vi "traceFileIO_writeToFile_multiple.vi"(0 "reference in":refnum<class "OSA.lvclass">, 1 "Path":path, 3 "dataType":T2, 4 "traces idx":u32[](array[numeric]), 5 "error in (no error)":errorcluster, 7 "dialog (empty path)":bool) -> (13 "traces idx global":u32[](array[numeric]), 14 "reference out":refnum<class "OSA.lvclass">, 15 "actual path":path, 17 "cancelled":bool, 19 "error out":errorcluster)   [LabVIEW 2010, in "OSA.lvclass"]
doc: "Read several spectrum or interferogram data from traces, (FTSLib.dll allocated), and store in a single spf2 file."
uses:
  OSA.lvclass
  typeDef/acq_dataType.ctl
  typeDef/trace_properties_ui.ctl
  FTSLib.dll
  OSA20X_misc.lvlib
panel:
  in  "property":T1
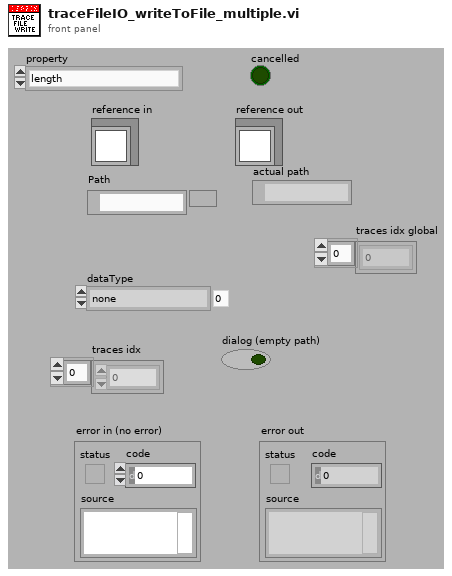
[diagram p1: front panel]
types:
  T1 = typedef "OSA.lvclass/trace_properties_ui.ctl" = enum16{"length", "type", "acquisitionMode", "xValueFormat", "date", "time", "averageNum", "smoothType", "igramSmoothType", "phaseCorrection", "apodisation", "__allocatedLengthI", "__allocatedLengthx", "adcBits", "sensitivityMode", "resolutionMode", "rollingAverage", "samplesPerReference", "air_measureOption", "interferogramProperty", "all_uiProperties"}
  T2 = typedef "OSA.lvclass/acq_dataType.ctl" = enum16{"none", "interferogram", "spectrum"}
  T3 = enum16{"SPC", "CSV", "SPF2", "TXT", "MAT_V5", "CSV_ZIP", "TXT_ZIP", "JCAMPDX"}
  T4 = typedef "OSA.lvclass/ObjectAttributes.ctl" = cluster{"Stop":bool, "dataType":T2, "spectrometerIdx":u16, "buffer size interferogram":i32, "interferogram":cluster{"new":bool, "plot_x_ min":sgl, "plot_x_max":sgl, "plot_y_min":sgl, "plot_y_max":sgl, "Graph Intrfrgrm":T5, "timeStamp":u32, "signal (%)":dbl, "traces":cluster{"idx":u32, "broadBand":bool, "monoChromatic":bool, "peakToPeakSignal":dbl, "peakToPeakPos":dbl}[], "traces idx last":i32}, "spectrum":cluster{"new":bool, "plot_x_min":sgl, "plot_x_max":sgl, "plot_unit_x":T6, "plot_unit_y":T7, "plot_y_min":sgl, "plot_y_max":sgl, "Graph Spectrum":T5, "timeStamp":u32, "X_VAL_OPTIONS":enum16{"MIN_MAX", "ARRAY"}, "traces":cluster{"idx":u32}[], "traces idx last":i32}, "Thorlabs_OSA_64.lvclass:queue_action.ctlqueue ref":refnum<queue>, "action":T8, "plot zoom step":dbl, "buffer semaphore":T9, "acq stopped":bool, "dataType active":T2, "temperature (degr C)":sgl, "pressure (hPa)":sgl, "rel humidity (%)":sgl, "settings":cluster{"resolution":T10, "sensitivity":T11, "Average":bool, "average nr":u32, "apodisation":T12, "acq delay (ms)":u32, "airMesure":T13, "wmtr on":bool, "intfgrm_smooth_width":u16, "intfgrm_smooth_nrOfPasses":u16, "intfgrm_smooth":T14, "phaseCorrection":T15, "zeroFill":u8, "spectr_smooth":T14, "spectr_smooth_width":u16, "spectr_smooth_nrOfPasses":u16, "resolution (/cm)":sgl, "REF wavelength, (nm)":dbl, "gain_idx":u16, "gainAuto":bool, "gain_relative":dbl, "PD sensitivity mode":T16, "PD senseMode implemented":bool, "SensorTemperature implemented":bool, "SensorPressure implemented":bool, "SensorHumidity implemented":bool}, "peaks position":sgl[], "peaks width":sgl[], "peaks height":sgl[], "peaks max nr":u32, "peaks latest nr":i32, "peaks new":bool, "power":dbl, "power new":bool, "path":string, "wavelength (WNr)":dbl, "wavelength new":bool, "buffer size spectrum":i32, "status":string, "VI reference":refnum<vi>, "funcPointer":u64, "libraryPointer":u64, "singleAcquisition":bool, "coherenceLength (cm)":dbl, "coherenceLength new":bool, "spectrometer model":string, "spectrometer serial nr":string, "peaks thld left":sgl[], "peaks thld right":sgl[], "coherenceLength error (cm)":dbl, "ADC bits":u16, "peaks position centroid":sgl[], "peaks height centroid":sgl[], "OSA series":T17, "channel index spectrum":u16, "spectrometer rangeLow, (/cm)":dbl, "spectrometer rangeHigh, (/cm)":dbl, "channel index interferogram":u16}
  T5 = typedef "OSA.lvclass/graph_intensity.ctl" = refnum<vi>
  T6 = typedef "OSA.lvclass/spectrum_x_unit.ctl" = enum16{"wavenr/cm", "THz", "eV", "nm_air", "nm_vac"}
  T7 = typedef "OSA.lvclass/y_unit.ctl" = enum16{"ADC counts", "dBm pwr absolute", "dBm pwr density", "mW pwr absolute", "mW pwr density"}
  T8 = typedef "OSA.lvclass/queue_action.ctl" = enum16{"none", "stop", "GUI_plotInterferogram", "GUI_plotSpectrum", "GUI_plotInterferogramRescale", "GUI_plotSpectrumRescale", "GUI_plotInterferogramReset", "GUI_plotSpectrumReset", "GUI_plotInterferogramAutoScaleY", "GUI_plotSpectrumAutoScaleY", "GUI_plotInterferogramZoomOut", "GUI_plotSpectrumZoomOut", "GUI_plotInterferogramPane", "GUI_plotSpectrumPane", "GUI_plotInterferogramZoomMouse", "GUI_plotSpectrumZoomMouse", "ENVIRONMENT temperature", "ENVIRONMENT pressure", "MODE_resolution set", "MODE_resolution get", "MODE_sensitivity set", "MODE_sensitivity get", "MODE_PDTemperature set", "MODE_PDTemperature get", "REBOOT/RESET firmware", "ACQASYNC_acquireSingleSpectrum", "ACQASYNC_continuous start", "ACQASYNC_continuous stop\n", "ACQASYNC_get last interferogram", "ACQASYNC_get last spectrum", "ACQASYNC_get last waveNr", "ACQOPT_interferogram smoothing set", "ACQOPT_interferogram smoothing get", "ACQOPT_spectrum smoothing set", "ACQOPT_spectrum smoothing get", "ACQOPT_apodisation type set", "ACQOPT_apodisation type get", "ACQOPT_phase correction type set", "ACQOPT_phase correction type get", "ACQOPT_acqIntervall_set", "ACQOPT_acqIntervall_get", "ACQOPT_average spectrum set", "ACQOPT_average spectrum get", "ACQOPT_rolling average set", "ACQOPT_rolling average get", "ACQOPT_zero fill factor set", "ACQOPT_zero fill factor get", "ACQOPT_cycle counting set", "ACQOPT_cycle counting get", "ACQOPT_air measure option set", "ACQOPT_air measure option get", "ACQOPT_gainLevel auto get", "ACQOPT_gainLevel auto set", "ACQOPT_gainLevel get", "ACQOPT_gainLevel set", "ACQOPT_getAll", "INSTRUMENT_PROPERTY_range_WaveNr_min", "INSTRUMENT_PROPERTY_range_WaveNr_max", "INSTRUMENT_PROPERTY_reference_wavelength_cm^-1", "INSTRUMENT_PROPERTY_samplesPerRefPeriod", "INSTRUMENT_PROPERTY_resolution_waveNrPercm", "INSTRUMENT_PROPERTY_availableGainLevels", "INSTRUMENT_PROPERTY_status", "CONVERT", "ANALYSE_POWER", "ANALYSE_PEAKS", "ANALYSE_WAVELENGTH", "ANALYSE_SPECTRUM", "ANALYSE_INTERFEROGRAM", "ANALYSE_COHERENCE_LENGTH", "MATH", "MATH_power", "MATH_peaks", "FILE", "miscellaneous"}
  T9 = typedef "Semaphore RefNum" = refnum<k1>
  T10 = typedef "OSA.lvclass/resolution.ctl" = enum16{"low", "high"}
  T11 = typedef "OSA.lvclass/sensitivityMode.ctl" = enum16{"low", "low medium", "high medium", "high"}
  T12 = typedef "OSA.lvclass/apodisation.ctl" = enum16{"NONE", "NORTON_BEER_WEAK", "NORTON_BEER_MEDIUM", "NORTON_BEER_STRONG", "TRIANGULAR", "COSINE", "HANN", "HAMMING", "BLACKMANHARRIS3", "BLACKMANHARRIS4", "GAUSSIAN"}
  T13 = typedef "OSA.lvclass/airMeasure.ctl" = enum16{"TEMPERATURE", "PRESSURE"}
  T14 = typedef "OSA20X_misc.lvlib/interferogram_smoothing.ctl" = enum16{"NONE", "BINOMIAL", "SAVITSKY_GOLAY", "FOURIER", "MOVING_AVERAGE", "GAUSSIAN"}
  T15 = typedef "OSA.lvclass/phaseCorrection.ctl" = enum16{"NONE", "MERTZ", "FORMAN", "MERTZ_FILE", "FORMAN_FILE", "FUTURE COMP."}
  T16 = typedef "OSA20X_misc.lvlib/PDTemperatureMode.ctl" = enum16{"cool: better sensitivity/noise floor", "warm: extended wl range"}
  T17 = typedef "OSA.lvclass/OSA_series.ctl" = enum16{"OSA200", "OSA300", "UNKNOWN"}
  T18 = cluster{"idx":u32, "broadBand":bool, "monoChromatic":bool, "peakToPeakSignal":dbl, "peakToPeakPos":dbl}[]
  T19 = cluster{"property":string, "property value":u32}[]
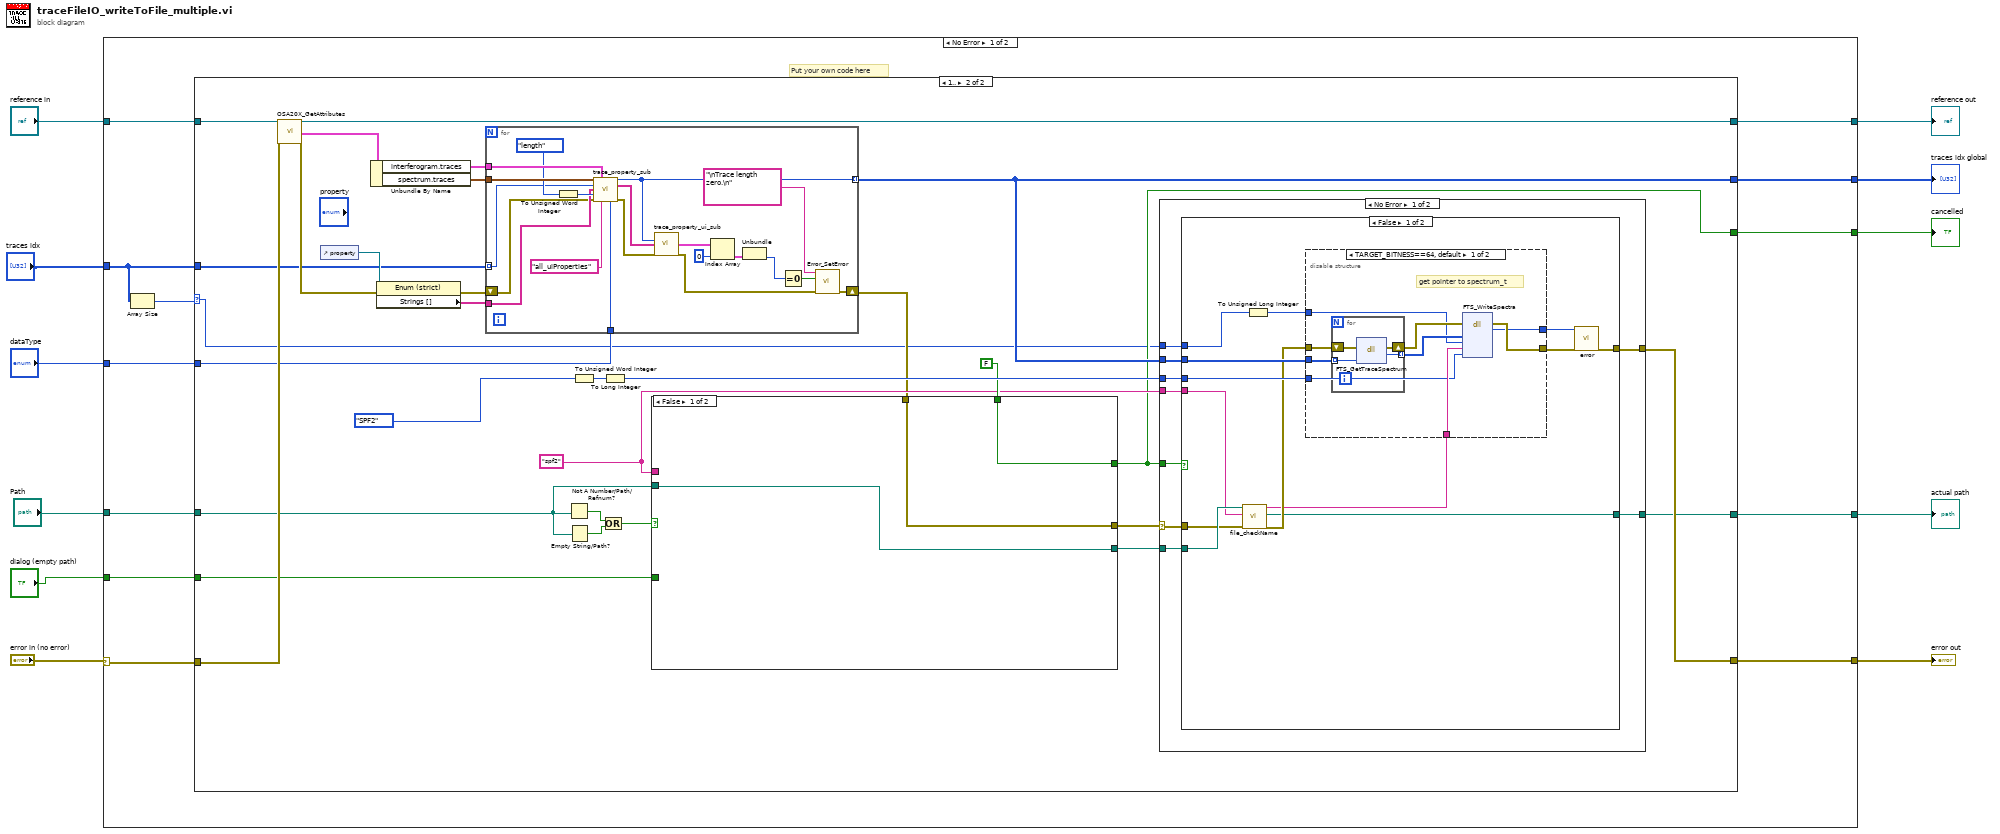
[diagram p0: block diagram]
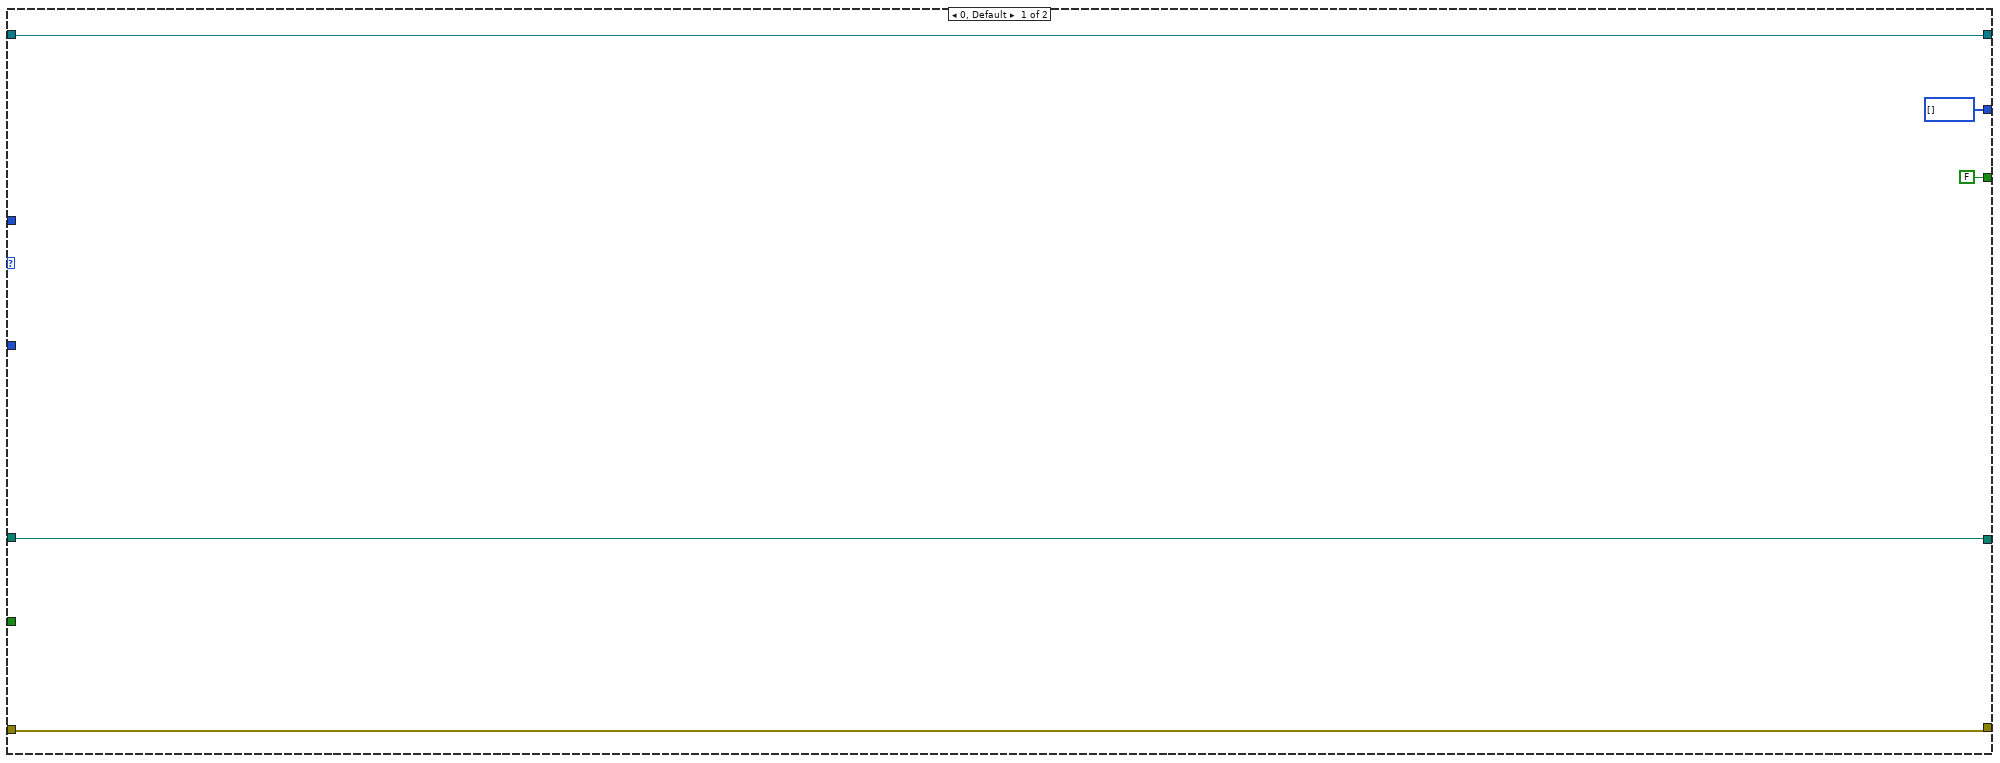
[diagram p2: hidden frame]
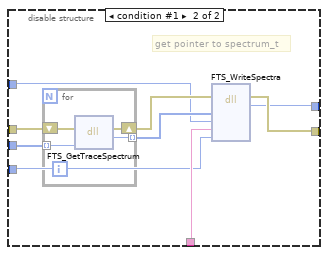
[diagram p3: hidden frame]
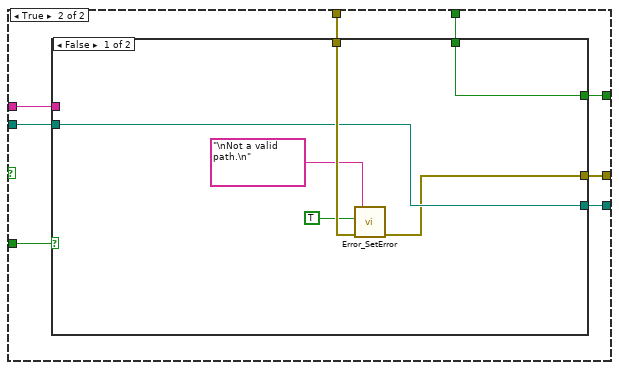
[diagram p6: hidden frame]
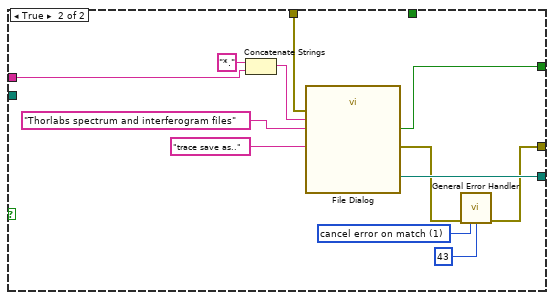
[diagram p7: hidden frame]
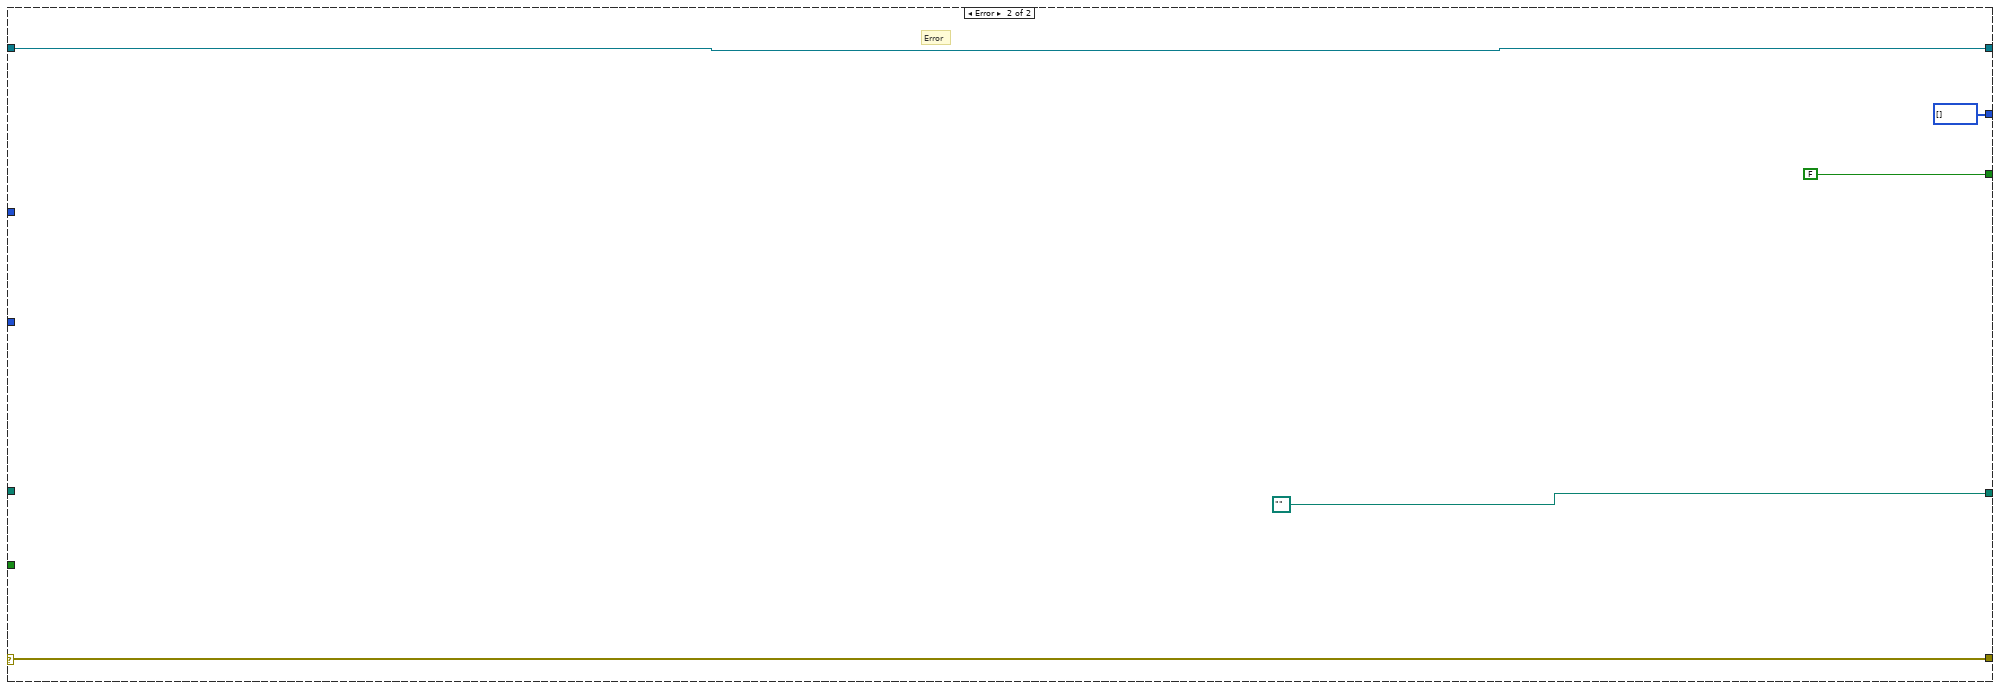
[diagram p8: hidden frame]
diagram:
  n1 = case shown="No Error" "error in (no error)" {
    selector: "error in (no error)" -> [w23 w164]
    tunnel: [w19 w164] -> w11
    tunnel: "reference in" -> [w22 w163]
    tunnel: [w21 w163] -> w8
    tunnel: "dataType" -> [w15 _]
    tunnel: "traces idx" -> [w12 _]
    tunnel: [w16 u32[] []] -> w6
    tunnel: "Path" -> [w20 _]
    tunnel: "dialog (empty path)" -> [w18 _]
    tunnel: [w17 path "" ("selected path")] -> w3
    tunnel: [w14 FALSE ("cancelled")] -> w2
    frame No Error {
      # "Put your own code here"
      n2 = Array Size(array=w12) -> (size(s)=w13:i32)
      n3 = case shown="1.." w13 {
        selector: w13 -> [_ w29]
        tunnel: w23 -> [w27 w57]
        tunnel: w22 -> [w26 w56]
        tunnel: [w26 w55] -> w21
        tunnel: w20 -> [w28 w51]
        tunnel: [w27 w50] -> w19
        tunnel: w18 -> [_ w49]
        tunnel: [w28 w42] -> w17
        tunnel: [u32[] [] w41] -> w16
        tunnel: w15 -> [_ w40]
        tunnel: [FALSE ("cancelled") w34] -> w14
        tunnel: w12 -> [_ w30]
        frame 0, Default {
        }
        frame 1.. {
          w43 = "spf2" ("pattern (all files)")
          n4 = call "OSA20X_GetAttributes.vi"("reference in"=w56, "error in (no error)"=w57) -> ("reference out"=w55:refnum<class "OSA.lvclass">, "Data"=w58:T4, "error out"=w36:errorcluster)  [unwired: 14 in, 1 out]
          n5 = control-ref of="property"() -> (w37:refnum<vi>)
          n6 = Unbundle By Name(w58) -> ("interferogram.traces"=w38:T18, "spectrum.traces"=w39:cluster{"idx":u32}[])
          n7 = property class="Enum (strict)"(reference=w37, error in=w36) -> (error out=w33:errorcluster, "Strings []"=w35:string[])  [unwired: 1 out]
          n8 = for {
            tunnel: [w73] -> w41 mode=indexing
            tunnel: w40 -> [w72]
            tunnel: w39 -> [w71]
            tunnel: w38 -> [w70]
            tunnel: w35 -> [w62]
            shift-right: [w60] -> w32
            shift-left: w33 -> [w61]
            tunnel: w30 -> [w59] mode=indexing
            n9 = To Unsigned Word Integer(number=trace_properties_ui."length" ("property")) -> (unsigned 16bit integer=w74:u16)
            n10 = call "trace_property_sub.vi"("traces_spectrum"=w71, "traces_interferogram"=w70, "trace idx"=w59, "Strings enum"=w62, "Value enum"=w74, "error in (no error)"=w61, "all string"="all_uiProperties", "dataType"=w72) -> ("global trace idx"=w73:u32, "parameter names"=w77:string[], "error out"=w69:errorcluster)  [unwired: 4 in, 1 out]
            n11 = call "trace_property_ui_sub.vi"("trace idx global"=w73, "properties ui"=w77, "error in (no error)"=w69) -> ("properties"=w78:T19, "error out"=w63:errorcluster)  [unwired: 10 in, 1 out]
            n12 = Index Array(array=w78, index=0) -> (element=w66:cluster{"property":string, "property value":u32})
            n13 = Unbundle(w66) -> ("property value"=w65:u32)  [unwired: 1 out]
            n14 = Equal To 0?(x=w65) -> (x = 0?=w64:bool)
            n15 = call "Error_SetError.vi"("error in"=w63, "status (true)"=w64, "source(\"\")"="\nTrace length zero.\n" ("source(\"\")")) -> ("error out"=w60:errorcluster)  [unwired: 4 in]
          }
          n16 = Not A Number/Path/Refnum?(number/path/refnum=w51) -> (NaN/Path/Refnum?=w53:bool)
          n17 = Empty String/Path?(string/path=w51) -> (empty?=w54:bool)
          n18 = To Unsigned Word Integer(number=T3."SPF2" ("file format (SPF2)")) -> (unsigned 16bit integer=w46:u16)
          n19 = Or(x=w53, y=w54) -> (x .or. y?=w52:bool)
          n20 = To Long Integer(number=w46) -> (32bit integer=w45:i32)
          n21 = case shown="False" w52 {
            tunnel: w51 -> [w132 w137]
            tunnel: w49 -> [_ w141]
            tunnel: w32 -> [w133 w140]
            tunnel: [w131 w138] -> w34
            tunnel: [w132 w139] -> w47
            tunnel: [w133 w136] -> w48
            tunnel: FALSE ("cancelled") -> [w131 w135]
            tunnel: w43 -> [_ w134]
            frame False {
            }
            frame True {
              n22 = case shown="False" w141 {
                tunnel: w140 -> [w147 w157]
                tunnel: [w144 w156] -> w139
                tunnel: [w142 w155] -> w138
                tunnel: w137 -> [w144 _]
                tunnel: [w143 w149] -> w136
                tunnel: w135 -> [w142 _]
                tunnel: w134 -> [_ w148]
                frame False {
                  n23 = call "Error_SetError.vi"("error in"=w147, "status (true)"=TRUE, "source(\"\")"="\nNot a valid path.\n" ("source(\"\")")) -> ("error out"=w143:errorcluster)  [unwired: 4 in]
                }
                frame True {
                  w152 = 1 items=["no exception", "cancel error on match", "set error on match"] ("[exception action] (none:0)")
                  n24 = Concatenate Strings("*." ("string"), w148) -> (w153:string)
                  n25 = call "File Dialog"("prompt"="trace save as..", "error in"=w157, "pattern (all files)"=w153, "pattern label"="Thorlabs spectrum and interferogram files") -> ("selected path"=w156:path, "cancelled"=w155:bool, "error out"=w150:errorcluster)  [unwired: 8 in, 1 out]
                  n26 = call <vilib>:"General Error Handler.vi"("error in (no error)"=w150, "[exception action] (none:0)"=w152, "[exception code]"=43) -> ("error out"=w149:errorcluster)  [unwired: 8 in, 4 out]
                }
              }
            }
          }
          n27 = case shown="No Error" w48 {
            selector: w48 -> [w83 w130]
            tunnel: w41 -> [w87 _]
            tunnel: [w86 w130] -> w50
            tunnel: w34 -> [w82 _]
            tunnel: w47 -> [w85 w129]
            tunnel: w45 -> [w84 _]
            tunnel: w43 -> [w81 _]
            tunnel: [w80 w129] -> w42
            tunnel: w29 -> [w79 _]
            frame No Error {
              n28 = case shown="False" w82 {
                tunnel: w87 -> [w100 _]
                tunnel: [w99 w128] -> w86
                tunnel: w85 -> [w95 w127]
                tunnel: w84 -> [w98 _]
                tunnel: w83 -> [w94 w128]
                tunnel: w81 -> [w93 _]
                tunnel: [w90 w127] -> w80
                tunnel: w79 -> [w89 _]
                frame False {
                  n29 = call "file_checkName.vi"("path"=w95, "filename extension"=w93, "error in (no error)"=w94) -> ("path string out"=w91:string, "actual path"=w90:path, "error out"=w92:errorcluster)  [unwired: 13 in, 1 out]
                  n30 = To Unsigned Long Integer(number=w89) -> (unsigned 32bit integer=w88:u32)
                  n31 = disable-structure shown="TARGET_BITNESS==64, default" {
                    disable-tunnel: w100 -> [w105 w115]
                    disable-tunnel: w91 -> [w109 w120]
                    disable-tunnel: w92 -> [w104 w116]
                    disable-tunnel: [w108 w119] -> w97
                    disable-tunnel: [w107 w118] -> w96
                    disable-tunnel: w98 -> [w106 w114]
                    disable-tunnel: w88 -> [w101 w117]
                    frame condition #0 (active) {
                      # "get pointer to spectrum_t"
                      n32 = for {
                        tunnel: w105 -> [w113] mode=indexing
                        shift-right: [w111] -> w103
                        shift-left: w104 -> [w112]
                        tunnel: [w110] -> w102 mode=indexing
                        n33 = dll-call lib="FTSLib.dll" fn="FTS_GetTraceSpectrum"(error in=w112, "traceIdx"=w113) -> (error out=w111:errorcluster, "spectrum_t_pointer"=w110:u64)  [unwired: 3 in, 1 out]
                      }
                      n34 = dll-call lib="FTSLib.dll" fn="FTS_WriteSpectra"(error in=w103, "spectrum_t_pointer"=w102, "spectra_nr"=w101, "fileNameAndPath"=w109, "fileFormat"=w106) -> (error out=w108:errorcluster, "returnValue"=w107:u32)  [unwired: 6 in, 1 out]
                    }
                    frame condition #1 {
                      # "get pointer to spectrum_t"
                      n35 = for {
                        tunnel: w115 -> [w126] mode=indexing
                        shift-right: [w124] -> w122
                        shift-left: w116 -> [w125]
                        tunnel: [w123] -> w121 mode=indexing
                        n36 = dll-call lib="FTSLib.dll" fn="FTS_GetTraceSpectrum"(error in=w125, "traceIdx"=w126) -> (error out=w124:errorcluster, "spectrum_t_pointer"=w123:u32)  [unwired: 3 in, 1 out]
                      }
                      n37 = dll-call lib="FTSLib.dll" fn="FTS_WriteSpectra"(error in=w122, "spectrum_t_pointer"=w121, "spectra_nr"=w117, "fileNameAndPath"=w120, "fileFormat"=w114) -> (error out=w119:errorcluster, "returnValue"=w118:u32)  [unwired: 6 in, 1 out]
                    }
                  }
                  n38 = call "error.vi"("result code"=w96, "error in (no error)"=w97) -> ("error out"=w99:errorcluster)  [unwired: 15 in, 2 out]
                }
                frame True {
                }
              }
            }
            frame Error {
            }
          }
        }
      }
    }
    frame Error {
      # "Error"
    }
  }
  "error out" <- w11
  "reference out" <- w8
  "traces idx global" <- w6
  "actual path" <- w3
  "cancelled" <- w2
